vi "Elevator.vi"(0 "Lower Limit Switch":bool, 2 "Driver Elevator Speed":dbl, 3 "Driver Invert":bool, 4 "Upper Limit Switch":bool, 5 "Give Driver Control?":bool, 6 "ELEV SEMSITIVITY":dbl, 7 "Lower":bool, 8 "Raise":bool, 9 "Override CoPilot":bool, 10 "Override Pilot":bool) -> ()   [LabVIEW 2015]
panel:
  out "one tick only":bool
  out "Go Over Limit Allowed":bool
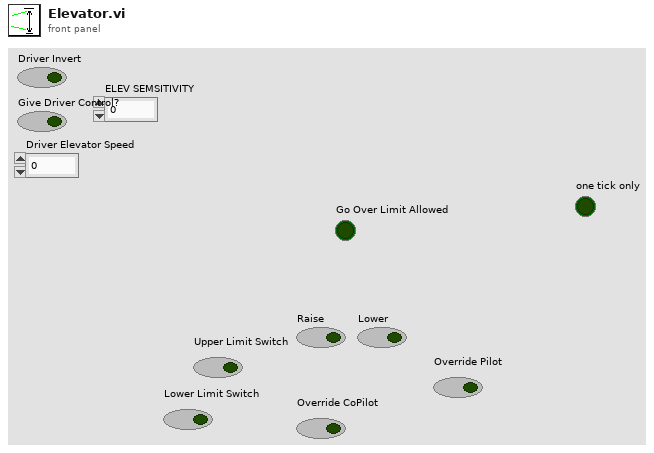
[diagram p1: front panel]
types:
  T1 = typedef "WPI_MotorControlDeviceRef.ctl" = cluster{"DeviceStatus":errorcluster, "Type":T2, "PWM":cluster{"PWM Channel":T3, "DeadBand":T4}, "CAN":cluster{"Device Number":u8, "Control Mode":T5, "Semaphore":T6, "Max Vout":dbl, "TalonSRX Control Mode":T7}, "Invert":bool}
  T2 = typedef "WPI_MotorControlType.ctl" = enum16{"PWM", "CAN", "CANTalonSRX"}
  T3 = typedef "FPGA_DIOPWMChannel.ctl" = enum8{"PWM 0", "PWM 1", "PWM 2", "PWM 3", "PWM 4", "PWM 5", "PWM 6", "PWM 7", "PWM 8", "PWM 9", "PWM MXP 0", "PWM MXP 1", "PWM MXP 2", "PWM MXP 3", "PWM MXP 4", "PWM MXP 5", "PWM MXP 6", "PWM MXP 7", "PWM MXP 8", "PWM MXP 9", "Invalid"}
  T4 = typedef "WPI_PWMDeadband.ctl" = cluster{"Name":string, "maxPositivePwm":i32, "minPositivePwm":i32, "centerPwm":i32, "maxNegativePwm":i32, "minNegativePwm":i32, "angularRange":u16}
  T5 = typedef "WPI_CANJaguar_ControlMode.ctl" = enum8{"Percent VBus", "Current", "Speed", "Position", "Voltage"}
  T6 = typedef "Semaphore RefNum" = refnum<k1>
  T7 = typedef "WPI_CANTalonSRX_APIControlMode.ctl" = enum8{"Percent VBus", "Speed", "Position", "Slave", "Unchanged / Invalid", "Voltage Compensation", "Current", "Motion Profile"}
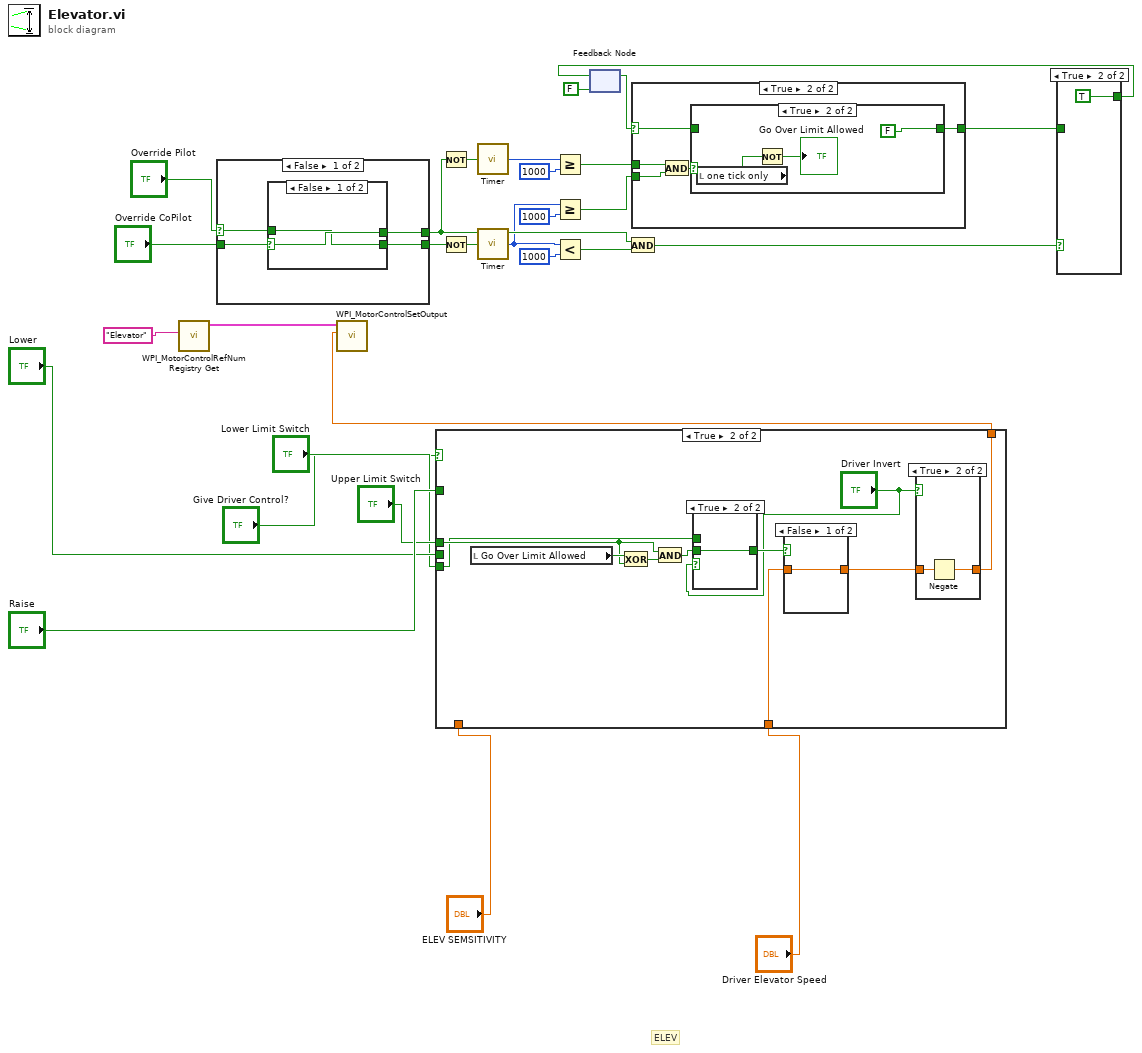
[diagram p0: block diagram]
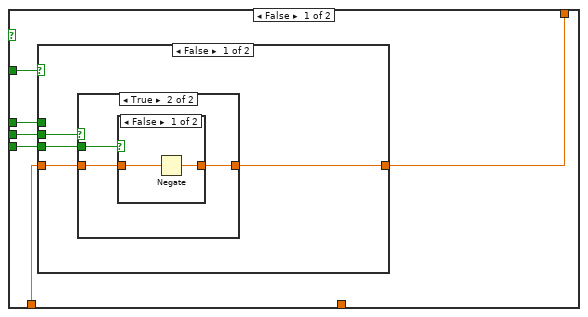
[diagram p2: hidden frame]
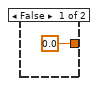
[diagram p3: hidden frame]
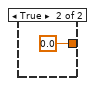
[diagram p4: hidden frame]
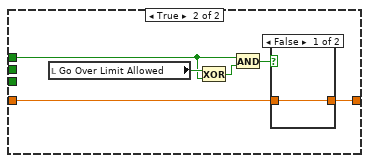
[diagram p5: hidden frame]
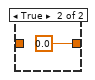
[diagram p6: hidden frame]
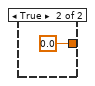
[diagram p9: hidden frame]
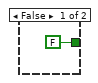
[diagram p10: hidden frame]
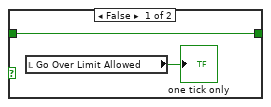
[diagram p11: hidden frame]
diagram:
  # "ELEV"
  n1 = call <vilib>:"WPI_MotorControlRefNum Registry Get.vi"("refnum name"="Elevator") -> ("MotorControlDevRef"=w4:T1)  [unwired: 9 in, 1 out]
  n2 = case shown="False" "Override Pilot" {
    selector: "Override Pilot" -> [w30 w39]
    tunnel: "Override CoPilot" -> [w33 w38]
    tunnel: [w32 w38] -> w19
    tunnel: [w31 w39] -> w14
    frame False {
      n3 = case shown="False" w33 {
        selector: w33 -> [w35 w37]
        tunnel: [w35 w36] -> w32
        tunnel: [w34 w37] -> w31
        tunnel: w30 -> [w34 w36]
        frame False {
        }
        frame True {
        }
      }
    }
    frame True {
    }
  }
  n4 = case shown="True" "Give Driver Control?" {
    tunnel: "Raise" -> [w45 _]
    tunnel: "Lower" -> [w44 _]
    tunnel: "ELEV SEMSITIVITY" -> [w43 _]
    tunnel: [w42 w70] -> w7
    tunnel: "Upper Limit Switch" -> [w41 w72]
    tunnel: "Lower Limit Switch" -> [w40 w67]
    tunnel: "Driver Elevator Speed" -> [_ w69]
    frame False {
      n5 = case shown="False" w45 {
        tunnel: [w49 w62] -> w42
        tunnel: w44 -> [w48 _]
        tunnel: w43 -> [w47 w61]
        tunnel: w41 -> [_ w57]
        tunnel: w40 -> [w46 _]
        frame False {
          n6 = case shown="True" w48 {
            tunnel: [0.0 ("f") w52] -> w49
            tunnel: w47 -> [_ w53]
            tunnel: w46 -> [_ w51]
            frame False {
            }
            frame True {
              n7 = case shown="False" w51 {
                tunnel: [w54 0.0 ("f")] -> w52
                tunnel: w53 -> [w55 _]
                frame False {
                  n8 = Negate(x=w55) -> (-x=w54:dbl)
                }
                frame True {
                }
              }
            }
          }
        }
        frame True {
          n9 = local read "Go Over Limit Allowed"() -> (w59:bool)
          n10 = Exclusive Or(1:w57, 2:w59) -> (0:w60:bool)
          n11 = And(x=w57, y=w60) -> (x .and. y?=w58:bool)
          n12 = case shown="False" w58 {
            tunnel: [w63 0.0 ("f")] -> w62
            tunnel: w61 -> [w63 _]
            frame False {
            }
            frame True {
            }
          }
        }
      }
    }
    frame True {
      n13 = local read "Go Over Limit Allowed"() -> (w73:bool)
      n14 = Exclusive Or(1:w72, 2:w73) -> (0:w74:bool)
      n15 = And(x=w72, y=w74) -> (x .and. y?=w66:bool)
      n16 = case shown="True" "Driver Invert" {
        tunnel: [w75 w76] -> w68
        tunnel: w67 -> [w75 _]
        tunnel: w66 -> [_ w76]
        frame False {
        }
        frame True {
        }
      }
      n17 = case shown="False" w68 {
        tunnel: [w80 0.0 ("f")] -> w71
        tunnel: w69 -> [w80 _]
        frame False {
        }
        frame True {
        }
      }
      n18 = case shown="True" "Driver Invert" {
        tunnel: w71 -> [w77 w79]
        tunnel: [w77 w78] -> w70
        frame False {
        }
        frame True {
          n19 = Negate(x=w79) -> (-x=w78:dbl)
        }
      }
    }
  }
  n20 = call <vilib>:"WPI_MotorControlSetOutput.vi"("Output"=w7, "MotorControlDevRef"=w4) -> ()  [unwired: 7 in, 3 out]
  n21 = Not(x=w19) -> (.not. x?=w17:bool)
  n22 = Not(x=w14) -> (.not. x?=w8:bool)
  n23 = call "Timer.vi"("Start Timer"=w17) -> ("Time elapsed"=w18:u64)
  n24 = call "Timer.vi"("Start Timer"=w8) -> ("Time elapsed"=w11:u64)
  n25 = Greater Or Equal?(x=w18, y=u64 1000) -> (x >= y?=w24:bool)
  n26 = Greater Or Equal?(x=w11, y=u64 1000) -> (x >= y?=w23:bool)
  n27 = Less?(x=w11, y=u64 1000) -> (x < y?=w10:bool)
  n28 = feedback #1(FALSE) -> (w21:bool)
  n29 = And(x=w19, y=w10) -> (x .and. y?=w15:bool)
  n30 = case shown="True" w21 {
    selector: w21 -> [_ w83]
    tunnel: [FALSE w87] -> w22
    tunnel: w23 -> [_ w86]
    tunnel: w24 -> [_ w85]
    frame False {
    }
    frame True {
      n31 = And(x=w85, y=w86) -> (x .and. y?=w84:bool)
      n32 = case shown="True" w84 {
        tunnel: [w89 FALSE] -> w87
        tunnel: w83 -> [w89 _]
        frame False {
          n33 = local read "Go Over Limit Allowed"() -> (→"one tick only":bool)
        }
        frame True {
          n34 = local read "one tick only"() -> (w90:bool)
          n35 = Not(x=w90) -> (.not. x?=→"Go Over Limit Allowed":bool)
        }
      }
    }
  }
  n36 = case shown="True" w15 {
    tunnel: [w93 TRUE] -> w16
    tunnel: w22 -> [w93 _]
    frame False {
    }
    frame True {
    }
  }
  n37 = feedback-in #1(w16) -> ()
